vi "2_Trav_move_Sub.vi"(0 "Traverse Setups":string[](array[string]), 1 "Extra Command String":string, 2 "Work in Tunnel Coordinates?":T1, 3 "Home Z":T2, 5 "Traverse Positions":sgl[](array[numeric])=[0.0, 0.0, 0.0] format="%.2f", 7 "Display Error":bool=TRUE, 9 "Backlash Compensation?":bool=TRUE, 10 "Offset (Tun Cord) 1-2":sgl[](array[numeric]), 11 "Simulate/Run":T3, 12 "Row Number":i32=11, 13 "Currently on Point":i32=11, 14 "Last Part of Move?":bool=TRUE) -> (4 "Trav Position achieved":sgl[](array[numeric]) format="%.2f", 6 "Error from Traverse named":string, 15 "Error String":string)   [LabVIEW 2022 SP3]
uses:
  Controls/User_Specific_mode.ctl
  Controls/Home.ctl
  Controls/Tunnel_Coordinates.ctl
  Trav_mode.ctl
  Globals/Constants_global.vi
panel:
  out "Check Error":string
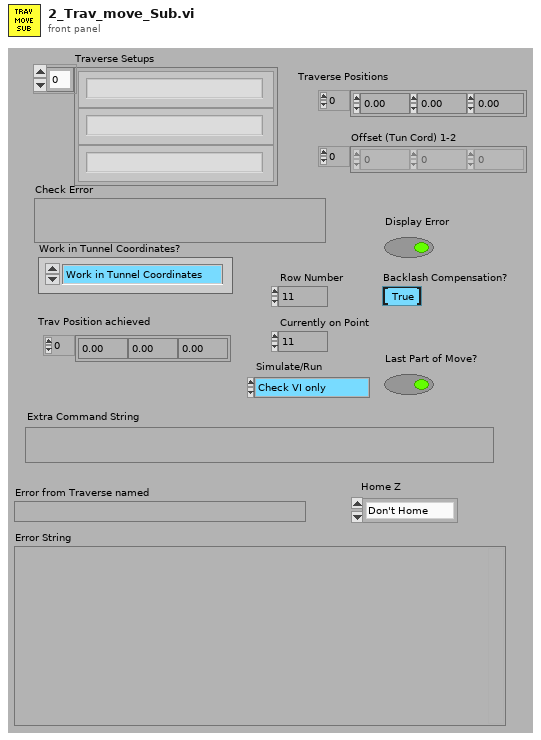
[diagram p1: front panel]
types:
  T1 = typedef "Tunnel_Coordinates.ctl" = enum16{"Work in Tunnel Coordinates", "Work in Model Coordinates"}
  T2 = typedef "Home.ctl" = enum16{"Don't Home", "Home  +X", "Home  -X", "Home  +Y", "Home  -Y", "Home  +Z", "Home  -Z"}
  T3 = typedef "User_Specific_mode.ctl" = enum16{"Check VI only", "Run VI"}
  T4 = typedef "Trav_mode.ctl" = enum16{"Move traverse", "Read traverse position", "Teach Position"}
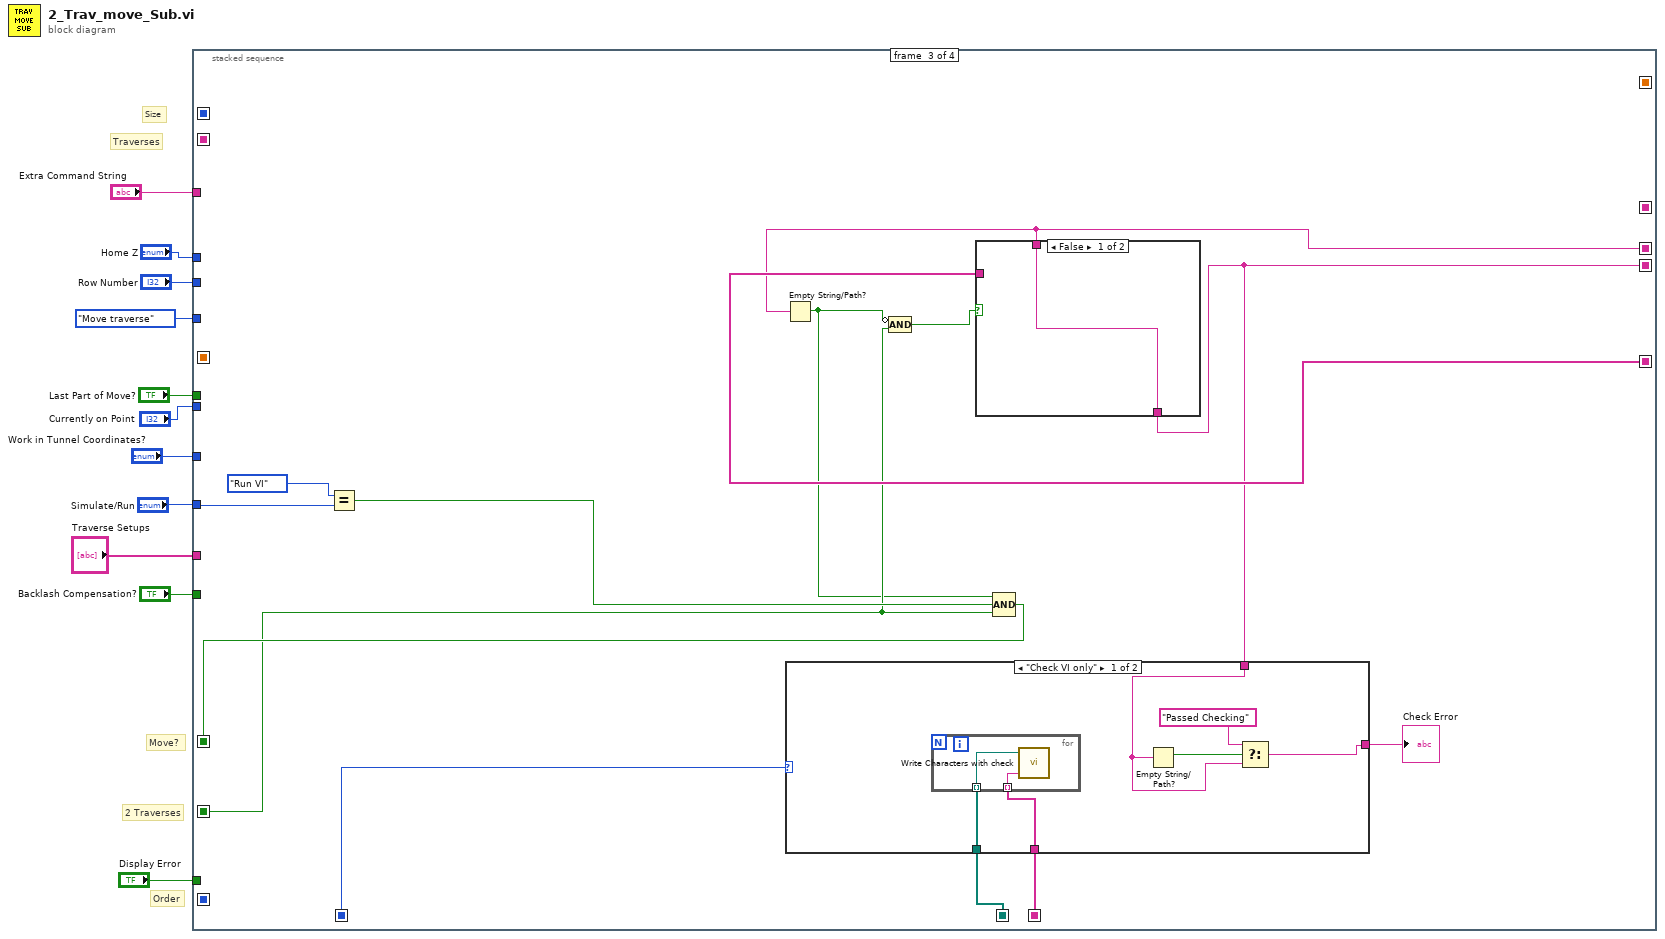
[diagram p0: block diagram]
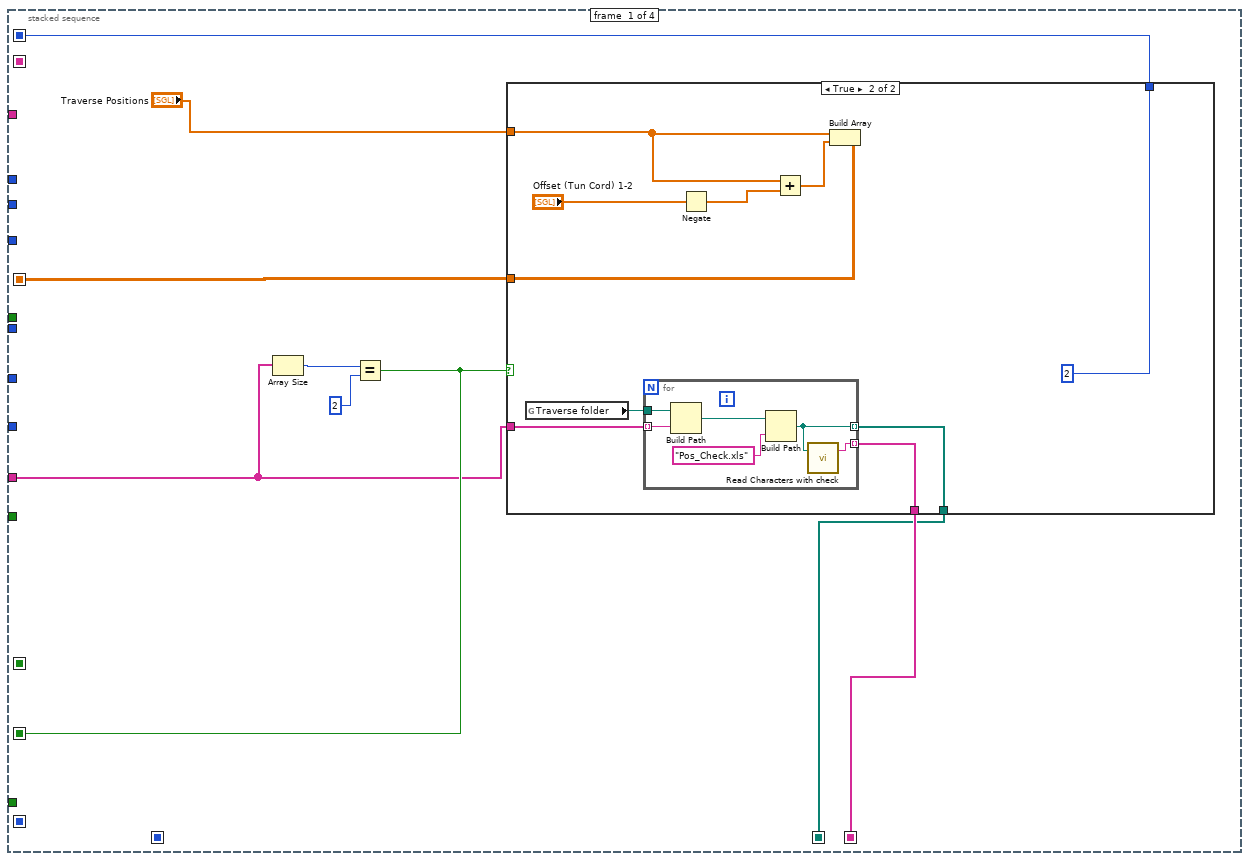
[diagram p2: hidden frame]
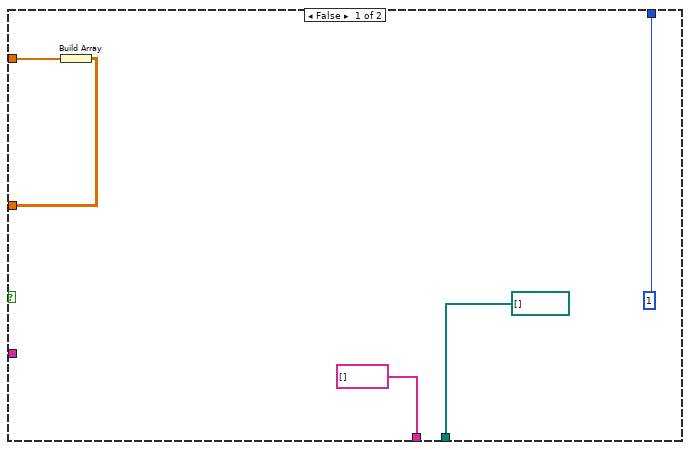
[diagram p3: hidden frame]
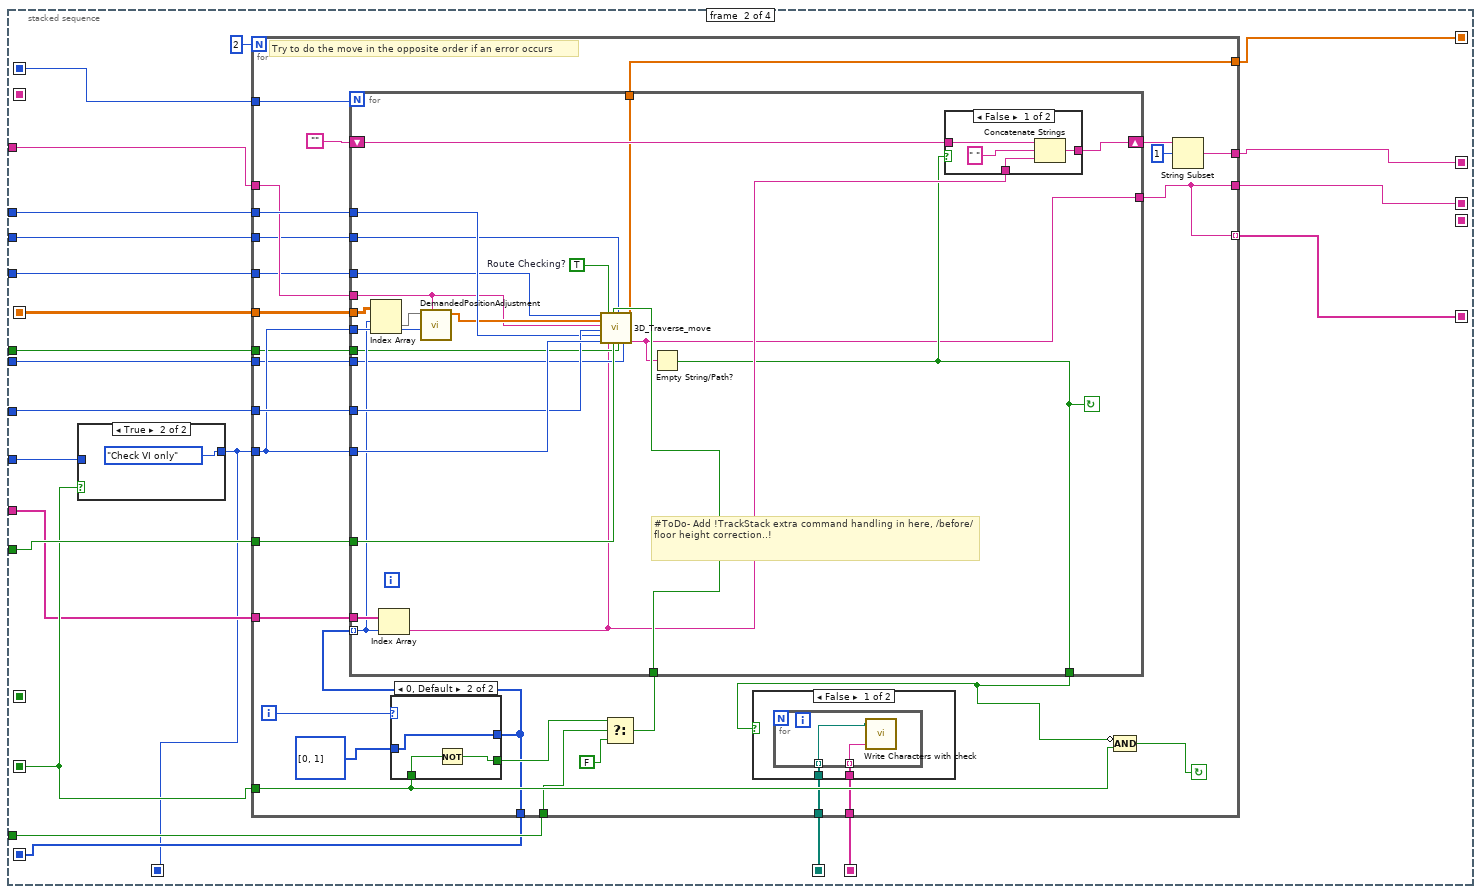
[diagram p4: hidden frame]
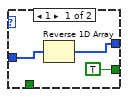
[diagram p7: hidden frame]
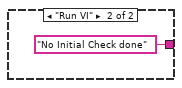
[diagram p9: hidden frame]
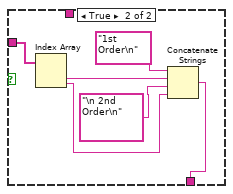
[diagram p10: hidden frame]
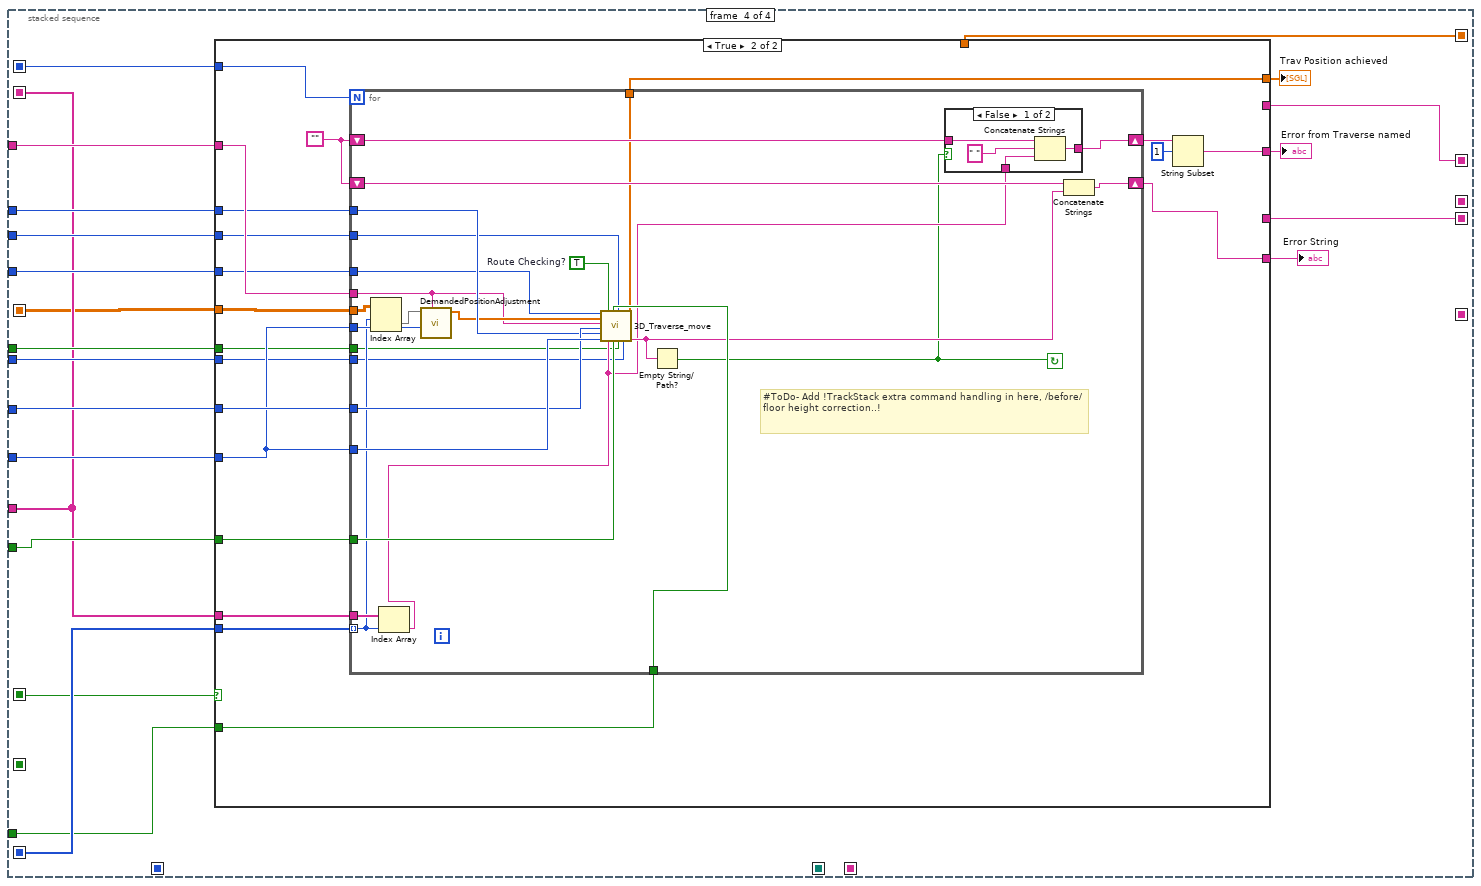
[diagram p11: hidden frame]
diagram:
  # "2 Traverses"
  # "Move?"
  # "Order"
  # "Size"
  # "Traverses"
  n1 = stacked-sequence {
    seq-local: [_ _ _ w166] -> [_ _ _ _]
    seq-local: [_ w60 _ _] -> [_ _ w147 _]
    seq-local: [_ w59 _ _] -> [_ _ w148 _]
    seq-local: [w16 _ _ _] -> [_ w58 _ w181]
    seq-local: [w18 _ _ _] -> [_ w56 w141 _]
    seq-local: [w17 _ _ _] -> [_ w55 w142 _]
    seq-local: [_ w50 _ _] -> [_ _ _ w170]
    seq-local: [_ w49 _ _] -> [_ _ _ w176]
    seq-local: [_ w47 _ _] -> [_ _ _ w172]
    seq-local: [_ _ w138 _] -> [_ _ _ w169]
    seq-local: [_ _ w143 _] -> [_ _ _ w167]
    seq-local: [w15 _ _ _] -> [_ w45 w137 _]
    seq-local: [_ w43 _ _] -> [_ _ w140 _]
    seq-local: [w12 _ _ _] -> [_ w42 _ w165]
    tunnel: "Extra Command String" -> [_ w64 _ w185]
    tunnel: "Work in Tunnel Coordinates?" -> [_ w62 _ w184]
    tunnel: "Simulate/Run" -> [_ w46 w146 w183]
    tunnel: "Backlash Compensation?" -> [_ w61 _ w182]
    tunnel: "Display Error" -> [_ w57 _ w175]
    tunnel: "Row Number" -> [_ w54 _ w180]
    tunnel: Trav_mode."Move traverse" ("Mode") -> [_ w53 _ w179]
    tunnel: "Last Part of Move?" -> [_ w52 _ w178]
    tunnel: "Currently on Point" -> [_ w51 _ w177]
    tunnel: "Home Z" -> [_ w48 _ w174]
    tunnel: "Traverse Setups" -> [w14 w44 _ w166]
    frame #0 {
      n2 = Array Size(array=w14) -> (size(s)=w20:i32)
      n3 = Equal?(x=w20, y=2) -> (x = y?=w15:bool)
      n4 = case shown="True" w15 {
        tunnel: w14 -> [_ w34]
        tunnel: [string[] [] w33] -> w18
        tunnel: [path[] [] w32] -> w17
        tunnel: [1 ("y") 2 ("y")] -> w16
        tunnel: "Traverse Positions" -> [w22 w28]
        tunnel: [w21 w27] -> w12
        frame False {
          n5 = Build Array(w22) -> (w21:sgl[][])
        }
        frame True {
          n6 = global read "Constants_global.vi" "Traverse folder"() -> (w35:path)
          n7 = for {
            tunnel: w35 -> [w39]
            tunnel: w34 -> [w38] mode=indexing
            tunnel: [w36] -> w33 mode=indexing
            tunnel: [w37] -> w32 mode=indexing
            n8 = Build Path(base path=w39, name or relative path=w38) -> (appended path=w40:path)
            n9 = Build Path(base path=w40, name or relative path="Pos_Check.xls" ("string")) -> (appended path=w37:path)
            n10 = call "Read Characters with check.vi"("file (use dialog)"=w37) -> ("Read String"=w36:string)  [unwired: 1 in, 1 out]
          }
          n11 = Negate(x="Offset (Tun Cord) 1-2") -> (-x=w29:sgl[])
          n12 = Add(x=w28, y=w29) -> (x+y=w30:sgl[])
          n13 = Build Array(w28, w30) -> (w27:sgl[][])
        }
      }
    }
    frame #1 {
      n14 = case shown="True" w45 {
        tunnel: [w65 User_Specific_mode."Check VI only" ("Simulate/Run")] -> w43
        tunnel: w46 -> [w65 _]
        frame False {
        }
        frame True {
        }
      }
      n15 = for {
        N: 2 -> [_]
        tunnel: w61 -> [w96]
        tunnel: w62 -> [w95]
        tunnel: [w91] -> w50
        tunnel: w48 -> [w90]
        tunnel: w42 -> [w88]
        tunnel: w43 -> [w87]
        tunnel: w44 -> [w86]
        tunnel: w58 -> [w85]
        tunnel: w64 -> [w89]
        tunnel: [w68] -> w60
        tunnel: w45 -> [w81]
        tunnel: [w68] -> w59 mode=indexing
        tunnel: w57 -> [w80]
        tunnel: w56 -> [w76]
        tunnel: w55 -> [w75]
        tunnel: [w74] -> w49
        tunnel: w54 -> [w73]
        tunnel: w53 -> [w72]
        tunnel: w52 -> [w71]
        tunnel: w51 -> [w70]
        tunnel: [w69] -> w47
        i -> [w84]
        stop <- w82 continue-if-true
        # "Try to do the move in the opposite order if an error occurs"
        n16 = case shown="0, Default" w84 {
          tunnel: [w102 w106] -> w74
          tunnel: i32[] [0, 1] -> [w103 w106]
          tunnel: [TRUE w104] -> w79
          tunnel: w81 -> [_ w105]
          frame 1 {
            n17 = Reverse 1D Array(array=w103) -> (reversed array=w102:i32[])
          }
          frame 0, Default {
            n18 = Not(x=w105) -> (.not. x?=w104:bool)
          }
        }
        n19 = Select(t=w79, s=w80, f=FALSE) -> (s? t:f=w77:bool)
        n20 = for {
          N: w85 -> [_]
          tunnel: w86 -> [w117]
          tunnel: w96 -> [w129]
          tunnel: w87 -> [w127]
          tunnel: w95 -> [w126]
          shift-right: [w125] -> w93
          shift-left: "" -> [w124]
          tunnel: w90 -> [w123]
          tunnel: w89 -> [w120]
          tunnel: w88 -> [w119]
          tunnel: w87 -> [w121]
          tunnel: w74 -> [w115] mode=indexing
          tunnel: w77 -> [w116]
          tunnel: [w108] -> w67
          tunnel: w73 -> [w114]
          tunnel: w72 -> [w113]
          tunnel: w71 -> [w112]
          tunnel: w70 -> [w111]
          tunnel: [w110] -> w69
          tunnel: [w107] -> w68
          stop <- w108 continue-if-true
          w128 = TRUE  # Route Checking?
          # "#ToDo- Add !TrackStack extra command handling in here, /before/ floor height correction..!"
          n21 = Index Array(array=w119, index (row)=w115) -> (element=w118:sgl[])  [unwired: 1 in]
          n22 = Index Array(array=w117, index=w115) -> (element=w109:string)
          n23 = call "DemandedPositionAdjustment.vi"("Extra Command String"=w120, "Simulate/Run"=w121, "Demanded Position"=w118) -> ("Adjusted Position"=w122:sgl[])  [unwired: 8 in]
          n24 = call "3D_Traverse_move.vi"("Mode"=w113, "Position"=w122, "Extra command String"=w120, "Work in Tunnel Coordinates"=w126, "Home"=w123, "Simulate/Run"=w127, "Route Checking?"=w128, "Traverse name"=w109, "Display Error"=w116, "Backlash Compensation?"=w129, "Row Number"=w114, "Last Part of Move?"=w112, "Currently on Point"=w111) -> ("Trav Position achieved"=w110:sgl[], "Error String"=w107:string)  [unwired: 3 in, 2 out]
          n25 = Empty String/Path?(string/path=w107) -> (empty?=w108:bool)
          n26 = case shown="False" w108 {
            tunnel: [w133 w134] -> w125
            tunnel: w124 -> [w132 w134]
            tunnel: w109 -> [w131 _]
            frame False {
              n27 = Concatenate Strings(w132, " " ("string"), w131) -> (w133:string)
            }
            frame True {
            }
          }
        }
        n28 = case shown="False" w67 {
          tunnel: w76 -> [w98 _]
          tunnel: w75 -> [w97 _]
          frame False {
            n29 = for {
              tunnel: w98 -> [w99] mode=indexing
              tunnel: w97 -> [w100] mode=indexing
              n30 = call "Write Characters with check.vi"("String to Write"=w99, "file (use dialog)"=w100) -> ()  [unwired: 2 in, 1 out]
            }
          }
          frame True {
          }
        }
        n31 = Compound Arithmetic op=AND(invert w67, w81) -> (w82:bool)
        n32 = String Subset(string=w93, offset (0)=1) -> (substring=w91:string)  [unwired: 1 in]
      }
    }
    frame #2 {
      n33 = Equal?(x=User_Specific_mode."Run VI" ("Simulate/Run"), y=w146) -> (x = y?=w144:bool)
      n34 = Empty String/Path?(string/path=w147) -> (empty?=w136:bool)
      n35 = Compound Arithmetic op=AND(invert w136, w137) -> (w135:bool)
      n36 = case shown="False" w135 {
        tunnel: [w158 w159] -> w138
        tunnel: w148 -> [_ w164]
        tunnel: w147 -> [w158 _]
        frame False {
        }
        frame True {
          n37 = Index Array(array=w164) -> (element #1=w162:string, element #2=w160:string)  [unwired: 2 in]
          n38 = Concatenate Strings("1st Order\n" ("string"), w162, "\n 2nd Order\n" ("string"), w160) -> (w159:string)
        }
      }
      n39 = case shown="\"Check VI only\"" w140 {
        tunnel: w142 -> [w154 _]
        tunnel: w141 -> [w153 _]
        tunnel: [w149 "No Initial Check done" ("Error String")] -> w139
        tunnel: w138 -> [w151 _]
        frame "Check VI only" {
          n40 = for {
            tunnel: w153 -> [w155] mode=indexing
            tunnel: w154 -> [w156] mode=indexing
            n41 = call "Write Characters with check.vi"("String to Write"=w155, "file (use dialog)"=w156) -> ()  [unwired: 2 in, 1 out]
          }
          n42 = Empty String/Path?(string/path=w151) -> (empty?=w152:bool)
          n43 = Select(t="Passed Checking", s=w152, f=w151) -> (s? t:f=w149:string)
        }
        frame "Run VI" {
        }
      }
      "Check Error" <- w139
      n44 = Compound Arithmetic op=AND(w136, w144, w137) -> (w143:bool)
    }
    frame #3 {
      n45 = case shown="True" w167 {
        tunnel: w185 -> [_ w208]
        tunnel: w184 -> [_ w207]
        tunnel: w183 -> [_ w206]
        tunnel: w182 -> [_ w205]
        tunnel: w166 -> [_ w204]
        tunnel: w165 -> [_ w203]
        tunnel: w181 -> [_ w202]
        tunnel: w180 -> [_ w201]
        tunnel: w179 -> [_ w200]
        tunnel: w178 -> [_ w199]
        tunnel: w177 -> [_ w198]
        tunnel: w176 -> [_ w194]
        tunnel: w175 -> [_ w193]
        tunnel: w174 -> [_ w192]
        tunnel: [w188 w191] -> w173
        tunnel: w172 -> [w188 _]
        tunnel: [w187 w190] -> w171
        tunnel: w170 -> [w187 _]
        tunnel: w169 -> [w186 _]
        tunnel: [w186 w189] -> w168
        frame False {
        }
        frame True {
          w197 = ""
          n46 = for {
            N: w202 -> [_]
            tunnel: w204 -> [w219]
            tunnel: w205 -> [w233]
            tunnel: w206 -> [w231]
            tunnel: w207 -> [w230]
            shift-right: [w228] -> w189
            shift-left: w197 -> [w229]
            shift-right: [w227] -> w196
            shift-left: w197 -> [w226]
            tunnel: w192 -> [w225]
            tunnel: w208 -> [w222]
            tunnel: w203 -> [w221]
            tunnel: w206 -> [w223]
            tunnel: w194 -> [w215] mode=indexing
            tunnel: w193 -> [w218]
            tunnel: w201 -> [w214]
            tunnel: w200 -> [w213]
            tunnel: w199 -> [w212]
            tunnel: w198 -> [w211]
            tunnel: [w210] -> w191
            stop <- w209 continue-if-true
            w232 = TRUE  # Route Checking?
            # "#ToDo- Add !TrackStack extra command handling in here, /before/ floor height correction..!"
            n47 = Index Array(array=w221, index (row)=w215) -> (element=w220:sgl[])  [unwired: 1 in]
            n48 = Index Array(array=w219, index=w215) -> (element=w216:string)
            n49 = call "DemandedPositionAdjustment.vi"("Extra Command String"=w222, "Simulate/Run"=w223, "Demanded Position"=w220) -> ("Adjusted Position"=w224:sgl[])  [unwired: 8 in]
            n50 = call "3D_Traverse_move.vi"("Mode"=w213, "Position"=w224, "Extra command String"=w222, "Work in Tunnel Coordinates"=w230, "Home"=w225, "Simulate/Run"=w231, "Route Checking?"=w232, "Traverse name"=w216, "Display Error"=w218, "Backlash Compensation?"=w233, "Row Number"=w214, "Last Part of Move?"=w212, "Currently on Point"=w211) -> ("Trav Position achieved"=w210:sgl[], "Error String"=w217:string)  [unwired: 3 in, 2 out]
            n51 = Empty String/Path?(string/path=w217) -> (empty?=w209:bool)
            n52 = case shown="False" w209 {
              tunnel: [w237 w238] -> w227
              tunnel: w226 -> [w236 w238]
              tunnel: w216 -> [w235 _]
              frame False {
                n53 = Concatenate Strings(w236, " " ("string"), w235) -> (w237:string)
              }
              frame True {
              }
            }
            n54 = Concatenate Strings(w229, w217) -> (w228:string)
          }
          n55 = String Subset(string=w196, offset (0)=1) -> (substring=w190:string)  [unwired: 1 in]
        }
      }
      "Trav Position achieved" <- w173
      "Error from Traverse named" <- w171
      "Error String" <- w168
    }
  }
